vi "IndexSampleData.vi"(11 "SampleData":string[][](array[string])) -> (1 "Y":dbl[](array[numeric]), 2 "SampleDataXYZ":cluster{"X":dbl[], "Y":dbl[], "Z":dbl[]}, 3 "X":dbl[](array[numeric]), 4 "Z":dbl[](array[numeric]))   [LabVIEW 2014, in "cyy.lvlib"]
uses:
  cyy.lvlib
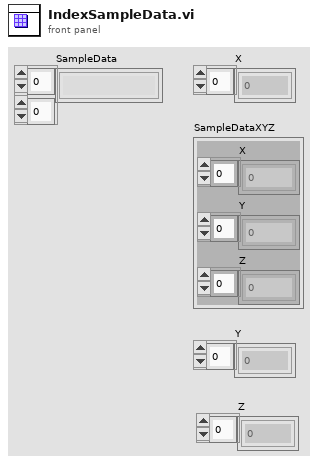
[diagram p1: front panel]
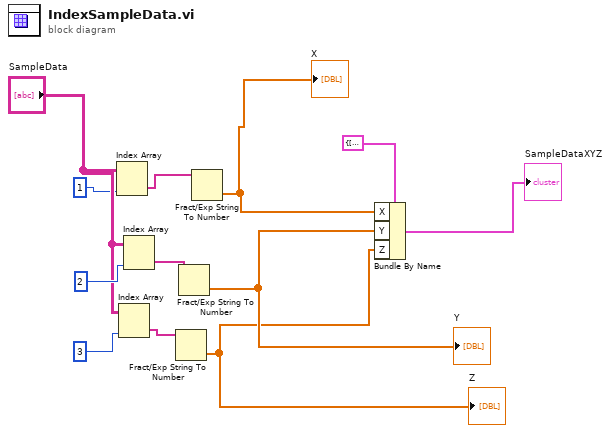
[diagram p0: block diagram]
diagram:
  n1 = Index Array(array="SampleData", index (col)=1) -> (element=w2:string[])  [unwired: 1 in]
  n2 = Index Array(array="SampleData", index (col)=3) -> (element=w7:string[])  [unwired: 1 in]
  n3 = Index Array(array="SampleData", index (col)=2) -> (element=w6:string[])  [unwired: 1 in]
  n4 = Fract/Exp String To Number(string=w7) -> (number=w9:dbl[])  [unwired: 3 in, 1 out]
  "Z" <- w9
  n5 = Fract/Exp String To Number(string=w6) -> (number=w10:dbl[])  [unwired: 3 in, 1 out]
  "Y" <- w10
  n6 = Fract/Exp String To Number(string=w2) -> (number=w8:dbl[])  [unwired: 3 in, 1 out]
  "X" <- w8
  n7 = Bundle By Name(cluster=cluster{"X":dbl[], "Y":dbl[], "Z":dbl[]} {"X"=[], "Y"=[], "Z"=[]}, "X"=w8, "Y"=w10, "Z"=w9) -> (→"SampleDataXYZ":cluster{"X":dbl[], "Y":dbl[], "Z":dbl[]})
